vi "ASK_Sync.vi"(1 "n":dbl, 6 "crc_num":i32, 7 "code_model":i32, 8 "error in (no error)":errorcluster caption="错误输入（无错误）", 9 "bitLen":i32, 10 "input_data":dbl[](array[numeric]) format="%#_13g", 11 "PathIn":path) -> (0 "error out":errorcluster caption="错误输出", 2 "output_data":dbl[](array[numeric]), 3 "PathOut":path)   [LabVIEW 2015]
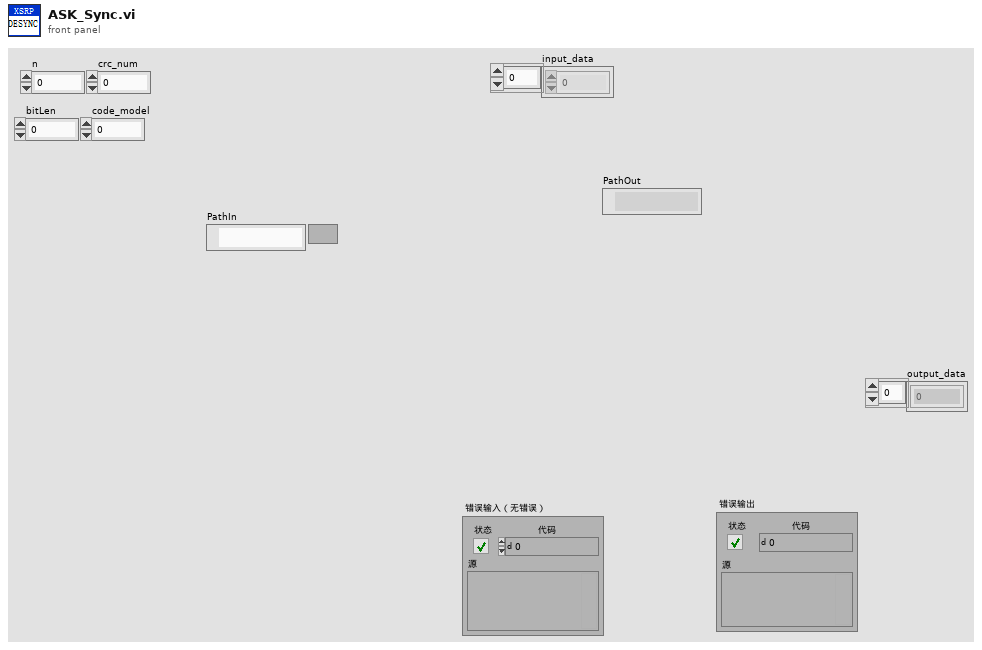
[diagram p1: front panel]
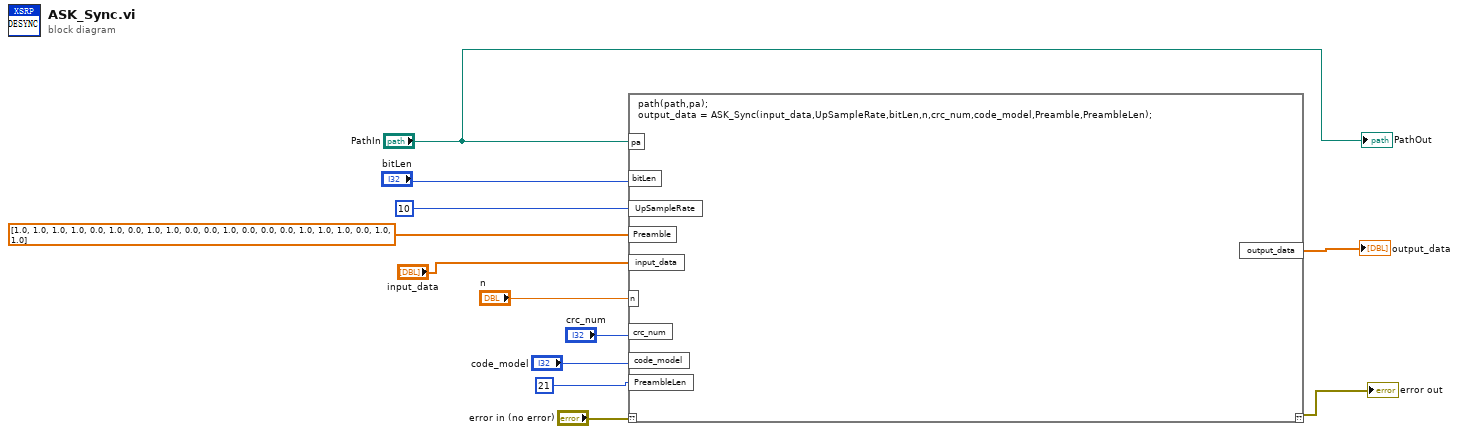
[diagram p0: block diagram]
diagram:
  n1 = script code="path(path,pa);\noutput_data = ASK_Sync(input_data,UpSampleRate,bitLen,n,crc_num,code_model,Preamble,PreambleLen);"("??"="error in (no error)", "pa"="PathIn", "input_data"="input_data", "n"="n", "UpSampleRate"=10, "bitLen"="bitLen", "crc_num"="crc_num", "code_model"="code_model", "Preamble"=dbl[] [1.0, 1.0, 1.0, 1.0, 0.0, 1.0, 0.0, 1.0, 1.0, 0.0, 0.0, 1.0, 0.0, 0.0, 0.0, 1.0, 1.0, 1.0, 0.0, 1.0, 1.0] ("数组"), "PreambleLen"=21) -> ("??"=→"error out":errorcluster, "output_data"=→"output_data":dbl[])
  "PathOut" <- "PathIn"
